vi "ReadAccessListTable.vi"(4 "error in (no error)":errorcluster, 7 "ADODB._Connection In":refnum<k7>) -> (0 "error out":errorcluster, 2 "SQL Results":string[][](table), 3 "ADODB._Connection Out":refnum<k7>)   [LabVIEW 2010]
doc: "This example opens a connection to a database specified by the Connection string (replace the DNS name with your database) and retrieves all the rows and columns from the table \"Table1\" (replace the SQL string with your own SQL query)."
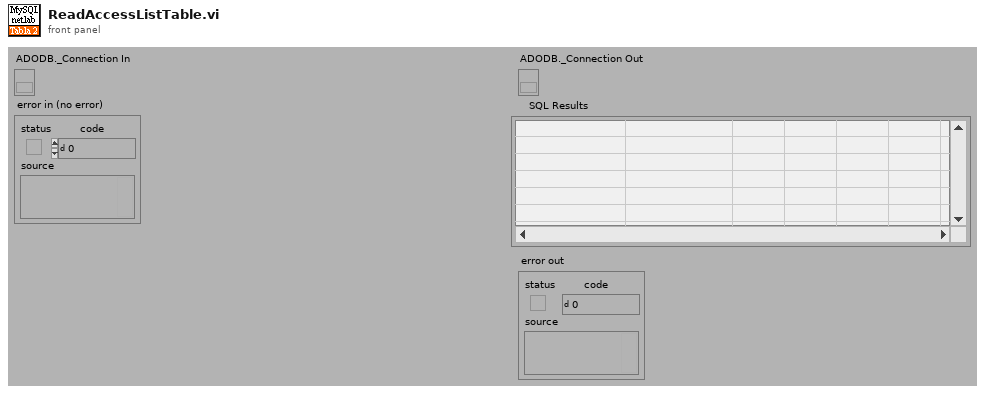
[diagram p1: front panel]
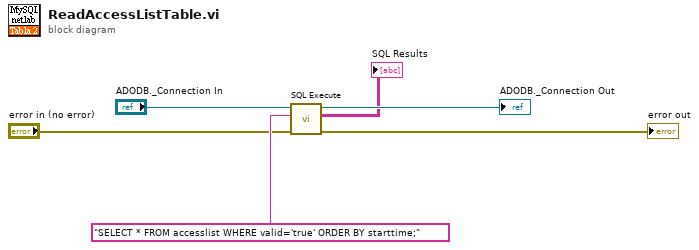
[diagram p0: block diagram]
diagram:
  n1 = call "SQL Execute.vi"("error in (no error)"="error in (no error)", "Command Text"="SELECT * FROM accesslist WHERE valid='true' ORDER BY starttime;", "ADODB._Connection In"="ADODB._Connection In") -> ("error out"=→"error out":errorcluster, "Data"=→"SQL Results":string[][], "ADODB._Connection Out"=→"ADODB._Connection Out":refnum<k7>)  [unwired: 1 in, 5 out]
